vi "Test Controller_Create.vi"(0 "reference in":refnum<class "Test Controller.lvclass">, 5 "error in (no error)":errorcluster) -> (14 "reference out":refnum<class "Test Controller.lvclass">, 19 "error out":errorcluster)   [LabVIEW 2016, in "Test Controller.lvclass"]
doc: "Constructor."
uses:
  Test Controller.lvclass
  C:/Program Files (x86)/National Instruments/LabVIEW 2016/vi.lib/addons/_AddQ/G#Object/G#Object.lvclass
  <vilib>/addons/_AddQ/G#Object/G#Object.lvclass
  SYS/File Controller_llb/File Controller.lvclass
  GUI/GUI Controller_llb/GUI Controller.lvclass
  SYS/Devices Controller_llb/Devices Controller.lvclass
  SYS/Items Controller_llb/Items Controller.lvclass
  SYS/Notification Controller_class/Notification Controller.lvclass
  SYS/PartsTracking Controller_class/PartsTracking Controller.lvclass
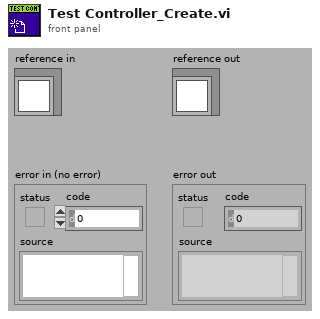
[diagram p1: front panel]
types:
  T1 = typedef "Test Controller.lvclass/ObjectAttributesRef.ctl" = refnum<data-value>
  T2 = typedef "Test Controller.lvclass/ClassAttributesRef.ctl" = refnum<data-value>
  T3 = typedef "Test Controller.lvclass/ClassAttributes.ctl" = cluster{"Dummy":bool, "test_controller_ref":refnum<class "Test Controller.lvclass">}
  T4 = typedef "Test Controller.lvclass/ObjectAttributes.ctl" = cluster{"MyAttribute":dbl, "Devices Controller_ref":refnum<class "Devices Controller.lvclass">, "File Controller_ref":refnum<class "File Controller.lvclass">, "Items Controller_ref":refnum<class "Items Controller.lvclass">, "GUI Controller_ref":refnum<class "GUI Controller.lvclass">, "NotificationController_ref":refnum<class "Notification Controller.lvclass">, "PartsTracking Controller_ref":refnum<class "PartsTracking Controller.lvclass">}
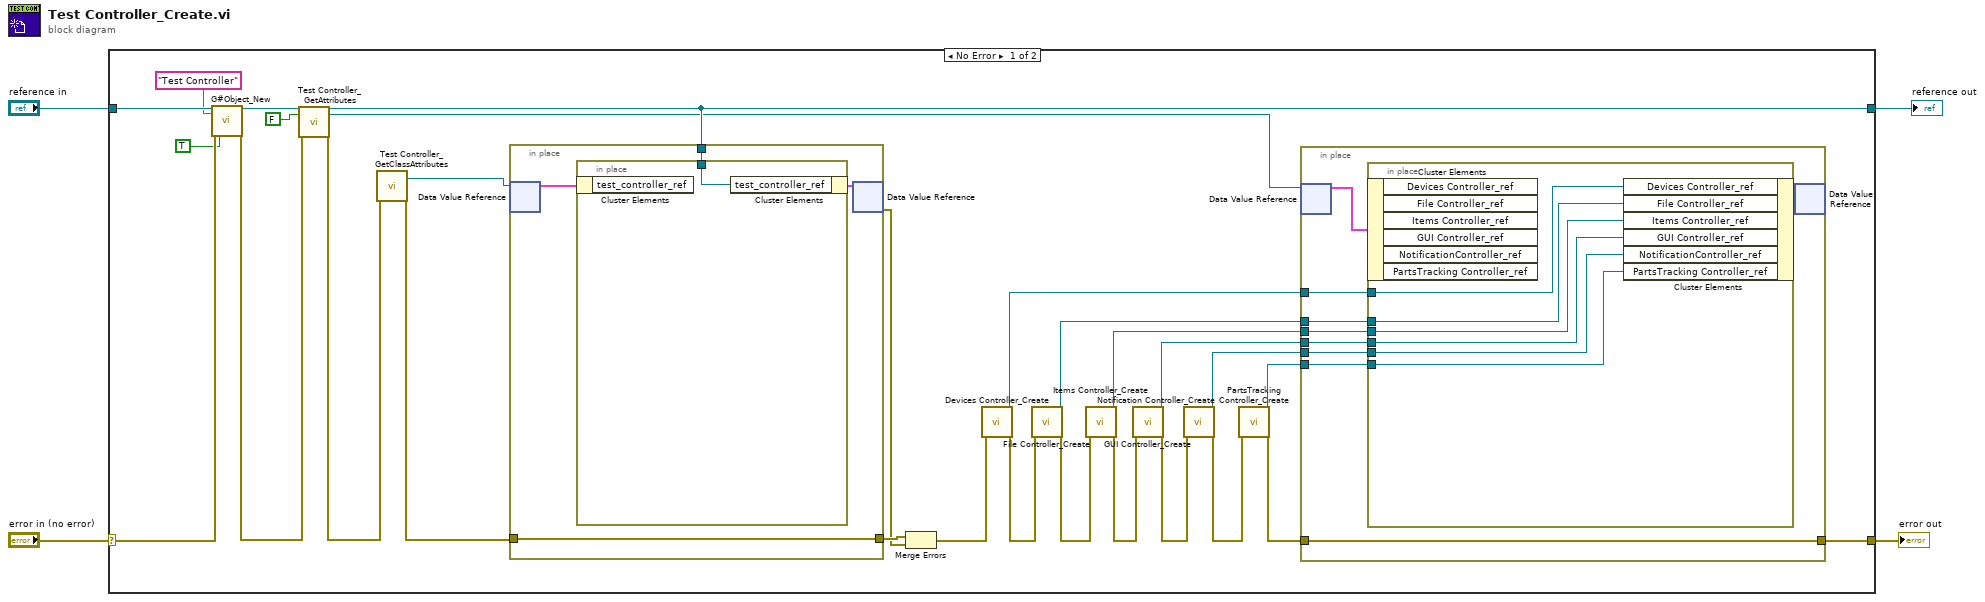
[diagram p0: block diagram]
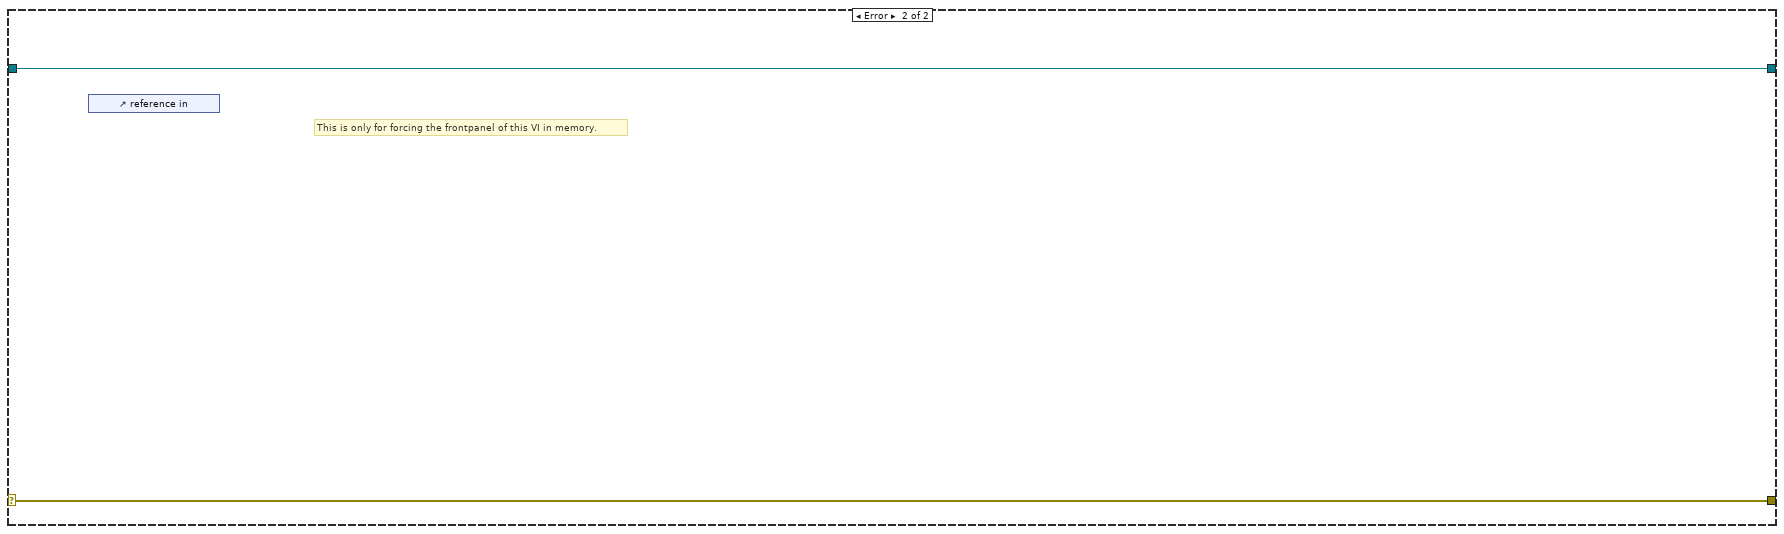
[diagram p2: hidden frame]
diagram:
  n1 = case shown="No Error" "error in (no error)" {
    selector: "error in (no error)" -> [w31 w54]
    tunnel: [w19 w54] -> w3
    tunnel: [w20 w53] -> w1
    tunnel: "reference in" -> [w32 w53]
    frame No Error {
      n2 = call <vilib>:"G#Object_New.vi"("reference in"=w32, "object name"="Test Controller", "error in (no error)"=w31, "user counter (T)?"=TRUE ("User Counter")) -> ("reference out"=w27:refnum<class "Test Controller.lvclass">, "error out"=w26:errorcluster)  [unwired: 13 in, 1 out]
      n3 = call "Test Controller_GetAttributes.vi"("reference in"=w27, "return data? (T)"=FALSE ("return data"), "error in (no error)"=w26) -> ("reference out"=w20:refnum<class "Test Controller.lvclass">, "attributes ref"=w18:T1, "error out"=w22:errorcluster)  [unwired: 13 in, 1 out]
      n4 = call "Test Controller_GetClassAttributes.vi"("error in (no error)"=w22) -> ("class attributes ref"=w23:T2, "error out"=w21:errorcluster)  [unwired: 15 in, 2 out]
      n5 = in-place {
        in-place-border: w21 -> [w49]
        in-place-border: [w49] -> w29
        in-place-border: w20 -> [w48]
        n6 = in-place-dvr #1(w23) -> (w50:T3)  [unwired: 1 out]
        n7 = in-place {
          in-place-border: w48 -> [w52]
          n8 = in-place-cluster #2(w50) -> ()  [unwired: 1 out]
          n9 = in-place-cluster #2("test_controller_ref"=w52) -> (w51:T3)
        }
        n10 = in-place-dvr #1(w51) -> (w28:errorcluster)  [unwired: 1 out]
      }
      n11 = Merge Errors(w29, w28) -> (w17:errorcluster)
      n12 = call "Devices Controller_Create.vi"("error in (no error)"=w17) -> ("error out"=w10:errorcluster, "reference out"=w16:refnum<class "Devices Controller.lvclass">)  [unwired: 9 in]
      n13 = call "File Controller_Create.vi"("error in (no error)"=w10) -> ("reference out"=w15:refnum<class "File Controller.lvclass">, "error out"=w9:errorcluster)  [unwired: 17 in]
      n14 = call "Items Controller_Create.vi"("error in (no error)"=w9) -> ("error out"=w8:errorcluster, "reference out"=w14:refnum<class "Items Controller.lvclass">)  [unwired: 9 in]
      n15 = call "GUI Controller_Create.vi"("error in (no error)"=w8) -> ("reference out"=w13:refnum<class "GUI Controller.lvclass">, "error out"=w7:errorcluster)  [unwired: 17 in]
      n16 = call "Notification Controller_Create.vi"("error in (no error)"=w7) -> ("reference out"=w12:refnum<class "Notification Controller.lvclass">, "error out"=w6:errorcluster)  [unwired: 17 in]
      n17 = call "PartsTracking Controller_Create.vi"("error in (no error)"=w6) -> ("reference out"=w11:refnum<class "PartsTracking Controller.lvclass">, "error out"=w5:errorcluster)  [unwired: 17 in]
      n18 = in-place {
        in-place-border: w5 -> [w39]
        in-place-border: [w39] -> w19
        in-place-border: w16 -> [w38]
        in-place-border: w15 -> [w37]
        in-place-border: w14 -> [w36]
        in-place-border: w13 -> [w35]
        in-place-border: w12 -> [w34]
        in-place-border: w11 -> [w33]
        n19 = in-place-dvr #3(w18) -> (w40:T4)  [unwired: 1 out]
        n20 = in-place {
          in-place-border: w38 -> [w47]
          in-place-border: w37 -> [w46]
          in-place-border: w36 -> [w45]
          in-place-border: w35 -> [w44]
          in-place-border: w34 -> [w43]
          in-place-border: w33 -> [w42]
          n21 = in-place-cluster #4(w40) -> ()  [unwired: 6 out]
          n22 = in-place-cluster #4("Devices Controller_ref"=w47, "File Controller_ref"=w46, "Items Controller_ref"=w45, "GUI Controller_ref"=w44, "NotificationController_ref"=w43, "PartsTracking Controller_ref"=w42) -> (w41:T4)
        }
        n23 = in-place-dvr #3(w41) -> ()  [unwired: 2 out]
      }
    }
    frame Error {
      # "This is only for forcing the frontpanel of this VI in memory."
      n24 = control-ref of="reference in"() -> ()  [unwired: 1 out]
    }
  }
  "error out" <- w3
  "reference out" <- w1
